vi "ReadEnc2.vi"() -> ()   [LabVIEW 2015]
uses:
  <instrlib>/Ion Motion Roboclaw/Ion Motion Roboclaw.lvlib
panel:
  out "Status":u8
  out "EncCnt":i32
  in  "Address":u8
  out "Valid":bool
  in  "stop":bool
  in  "COMPort":refnum<visa-resource-name>
  in  "baud rate (38400)":u32
  in  "error in (no error)":errorcluster
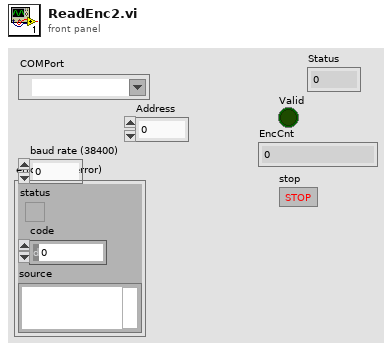
[diagram p1: front panel]
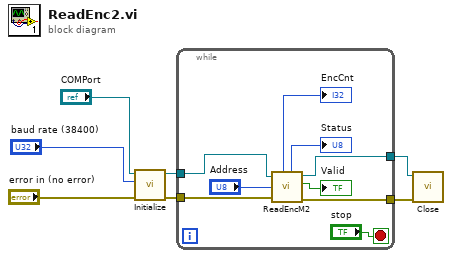
[diagram p0: block diagram]
diagram:
  n1 = call <instrlib>:"Initialize.vi"("error in (no error)"="error in (no error)", "baud rate (38400)"="baud rate (38400)", "COM port"="COMPort") -> ("error out"=w6:errorcluster, "VISA resource name out"=w7:refnum<visa-resource-name>)  [unwired: 7 in]
  n2 = while {
    tunnel: w7 -> [w15]
    tunnel: w6 -> [w14]
    tunnel: [w12] -> w5
    tunnel: [w13] -> w4
    stop <- "stop" stop-if-true
    n3 = call <instrlib>:"ReadEncM2.vi"("VISA Refnum in"=w15, "Address"="Address", "error in (no error)"=w14) -> ("EncCnt"=→"EncCnt":u32, "Status"=→"Status":u8, "VISA Refnum out"=w12:refnum<visa-resource-name>, "Valid"=→"Valid":bool, "error out"=w13:errorcluster)  [unwired: 3 in]
  }
  n4 = call <instrlib>:"Close.vi"("error in (no error)"=w4, "VISA resource name"=w5) -> ()  [unwired: 9 in, 1 out]
